vi "QueryServer_Event_Fire.vi"(7 "server id":i32, 8 "error in (no error)":errorcluster, 9 "status":i32, 10 "eventdata":string, 11 "gRPCid":T1) -> (0 "error out":errorcluster, 3 "gRPCid out":T1)   [LabVIEW 2019, in "labview-grpc-query-server.lvlib"]
uses:
  labview-grpc-query-server.lvlib
  gRPC interface/Server API/typeDefs/grpcId.ctl
  QueryServer_Event.ctl
  0bb59e7e-a377-41a5-9059-4bcd5e2faf60.vi
  <vilib>/Utility/error.llb/Error Cluster From Error Code.vi
  gRPC interface/gprc-lvsupport.lvlib
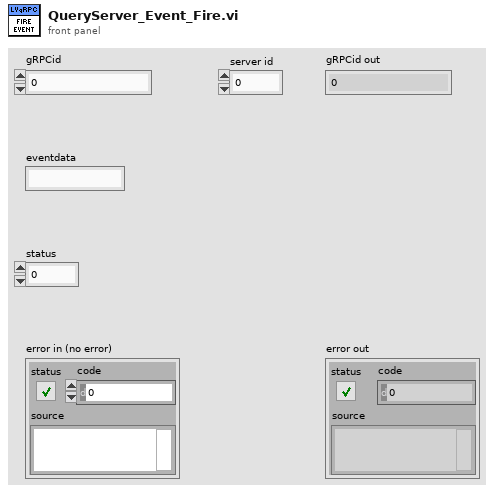
[diagram p1: front panel]
types:
  T1 = typedef "gprc-lvsupport.lvlib/grpcId.ctl" = u64
  T2 = typedef "labview-grpc-query-server.lvlib/QueryServer_Event.ctl" = cluster{"eventdata":string, "server id":i32, "status":i32}
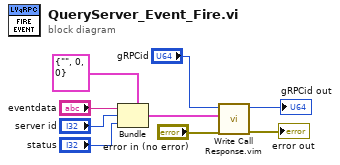
[diagram p0: block diagram]
diagram:
  n1 = Bundle(cluster=T2 {"eventdata"="", "server id"=0, "status"=0} ("ServerEvent"), "eventdata"="eventdata", "server id"="server id", "status"="status") -> (w5:T2)
  n2 = call "Write Call Response.vim"("error in (no error)"="error in (no error)", "Response Data"=w5, "gRPCid in"="gRPCid") -> ("error out"=→"error out":errorcluster, "gRPCid"=→"gRPCid out":T1)  [unwired: 7 in]
